vi "Parse Log File String.vi"(10 "Log File Chunk":u8[](array[numeric]), 11 "Remaining Bytes in":u8[](array[numeric])) -> (2 "Log FIle Lines":string[](array[string]), 3 "Remaining Bytes Out":u8[](array[numeric]))   [LabVIEW 2019]
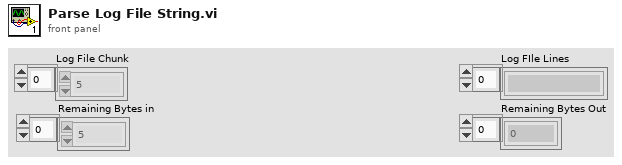
[diagram p1: front panel]
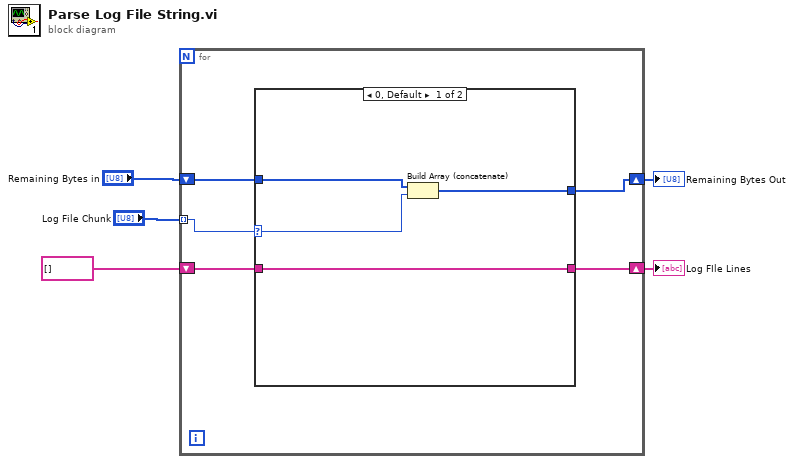
[diagram p0: block diagram]
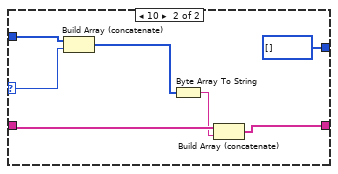
[diagram p2: hidden frame]
diagram:
  n1 = for {
    tunnel: "Log File Chunk" -> [w10] mode=indexing
    shift-right: [w8] -> w1
    shift-left: "Remaining Bytes in" -> [w9]
    shift-right: [w6] -> w2
    shift-left: string[] [] -> [w7]
    n2 = case shown="0, Default" w10 {
      selector: w10 -> [w13 w19]
      tunnel: w9 -> [w14 w20]
      tunnel: [w12 u8[] []] -> w8
      tunnel: w7 -> [w11 w17]
      tunnel: [w11 w15] -> w6
      frame 0, Default {
        n3 = Build Array (concatenate)(w14, w13) -> (w12:u8[])
      }
      frame 10 {
        n4 = Build Array (concatenate)(w20, w19) -> (w18:u8[])
        n5 = Byte Array To String(unsigned byte array=w18) -> (string=w16:string)
        n6 = Build Array (concatenate)(w17, w16) -> (w15:string[])
      }
    }
  }
  "Log FIle Lines" <- w2
  "Remaining Bytes Out" <- w1
